vi "Asynchronously Execute Python Optimization (Off-Grid).vi"(8 "error in":errorcluster, 10 "Stop Notifier":refnum<notifier>, 11 "Off-Grid in":refnum<class "Off-Grid.lvclass">) -> (0 "error out":errorcluster, 3 "Off-Grid out":refnum<class "Off-Grid.lvclass">)   [LabVIEW 2018, in "Off-Grid Actor.lvlib" / "Off-Grid.lvclass"]
uses:
  Off-Grid.lvclass
  C:/Users/Administrator/Desktop/LabVIEW EMS/Optimization/Generic Optimization Actor/Generic Optimization/Generic Optimization.lvclass
  Execute Python Optimization (Off-Grid).vi
  Global Variables/Global Variables.vi
  Generic Optimization Actor/Generic Optimization/Generic Optimization.lvclass
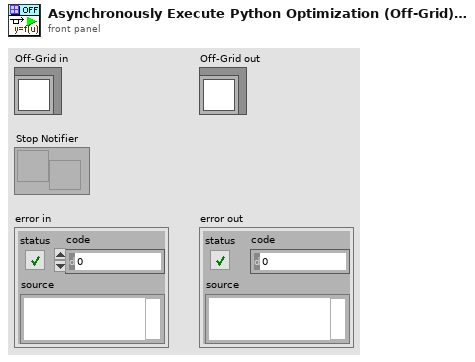
[diagram p1: front panel]
types:
  T1 = typedef "Optimization Type Selector.ctl" = enum16{"Invalid", "Single Phase", "Volttron"}
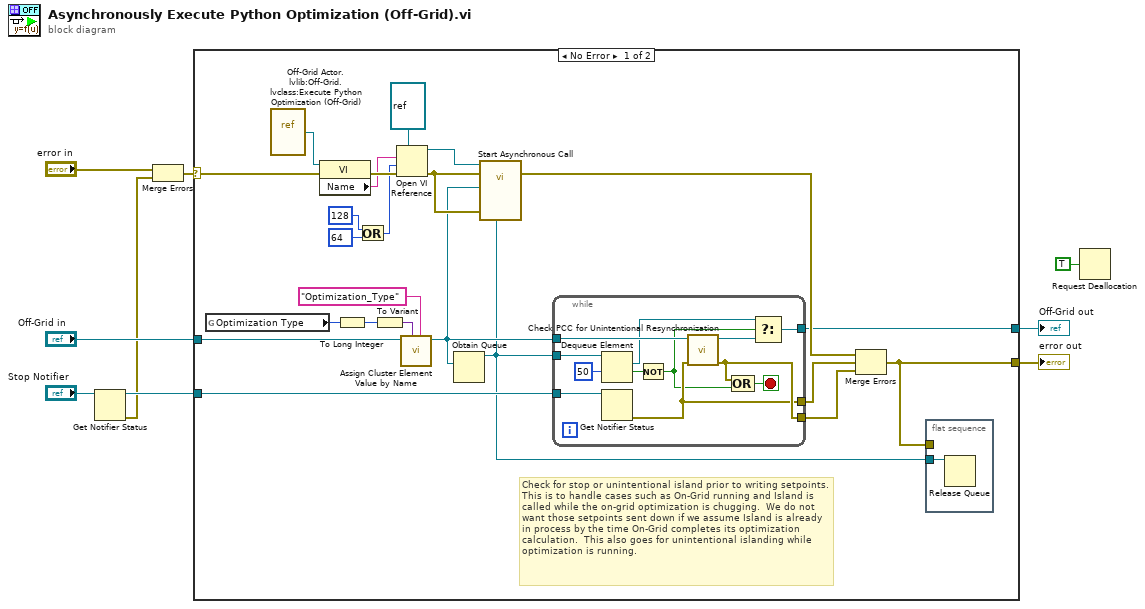
[diagram p0: block diagram]
diagram:
  n1 = Get Notifier Status(notifier="Stop Notifier") -> (notifier out=w5:refnum<notifier>, error out=w3:errorcluster)  [unwired: 1 in, 3 out]
  n2 = Merge Errors("error in", w3) -> (w2:errorcluster)
  n3 = case shown="No Error" w2 {
    selector: w2 -> [w32 w47]
    tunnel: w5 -> [w31 _]
    tunnel: [w30 w47] -> w9
    tunnel: "Off-Grid in" -> [w16 w46]
    tunnel: [w11 w46] -> w7
    frame No Error {
      # "Check for stop or unintentional island prior to writing setpoints.  This is to handle cases such as On-Grid running and Island is called while the on-grid optimization is chugging.  We do not want those setpoints sent down if we assume Island is already in process by the time On-Grid completes its optimization calculation.  This also goes for unintentional islanding while optimization is running."
      n4 = global read "Global Variables.vi" "Optimization Type"() -> (w28:T1)
      n5 = vi-ref "Off-Grid Actor.lvlib:Off-Grid.lvclass:Execute Python Optimization (Off-Grid).vi"() -> (w20:refnum<vi>)
      n6 = property class="VI"(reference=w20, error in=w32) -> (error out=w22:errorcluster, "Name"=w21:string)  [unwired: 1 out]
      n7 = To Long Integer(number=w28) -> (32bit integer=w29:i32)
      n8 = Or(x=128 ("options"), y=64 ("options")) -> (x .or. y?=w13:i32)
      n9 = To Variant(anything=w29) -> (Variant=w27:variant)
      n10 = Open VI Reference(type specifier VI Refnum (for type only)=refnum<vi> refnum, vi path=w21, options=w13, error in (no error)=w22) -> (vi reference=w25:refnum<vi>, error out=w23:errorcluster)  [unwired: 2 in]
      n11 = call "Assign Cluster Element Value by Name.vi"("Element Name"="Optimization_Type" ("Keyword Name"), "Value"=w27, "Generic Optimization"=w16) -> ("Generic Optimization out"=w12:refnum<class "Off-Grid.lvclass">)  [unwired: 7 in, 1 out]
      n12 = Obtain Queue(element data type=w12) -> (queue out=w10:refnum<queue>)  [unwired: 4 in, 2 out]
      n13 = call-by-ref "Start Asynchronous Call"(reference=w25, error in=w23, "Results Queue"=w10, "error in"=w23, "Off-Grid in"=w12) -> (error out=w24:errorcluster)  [unwired: 7 in, 3 out]
      n14 = while {
        tunnel: w31 -> [w45]
        tunnel: [w39] -> w17
        tunnel: w10 -> [w44]
        tunnel: w12 -> [w41]
        tunnel: [w38] -> w18
        tunnel: [w34] -> w11
        stop <- w40 stop-if-true
        n15 = Dequeue Element(queue=w44, timeout in ms (-1)=50) -> (element=w36:refnum<class "Off-Grid.lvclass">, timed out?=w42:bool)  [unwired: 1 in, 2 out]
        n16 = Get Notifier Status(notifier=w45) -> (error out=w38:errorcluster)  [unwired: 1 in, 4 out]
        n17 = Not(x=w42) -> (.not. x?=w37:bool)
        n18 = call "Check PCC for Unintentional Resynchronization.vi"("error in"=w38, "Off-Grid in"=w41) -> ("error out"=w39:errorcluster, "Off-Grid out"=w35:refnum<class "Off-Grid.lvclass">)  [unwired: 8 in]
        n19 = Compound Arithmetic op=OR(w39, w37) -> (w40:bool)
        n20 = Select(t=w36, s=w37, f=w35) -> (s? t:f=w34:refnum<class "Off-Grid.lvclass">)
      }
      n21 = Merge Errors(w24, w18, w17) -> (w30:errorcluster)
      n22 = flat-sequence {
        tunnel: w10 -> [w33]
        tunnel: w30 -> [_]
        frame #0 {
          n23 = Release Queue(queue=w33) -> ()  [unwired: 2 in, 3 out]
        }
      }
    }
    frame Error {
    }
  }
  "error out" <- w9
  "Off-Grid out" <- w7
  n24 = Request Deallocation(TRUE ("flag")) -> ()
